vi "Status set defs.vi"(8 "error in (no error)":errorcluster, 11 "MB_TCP in":refnum<class "MB_TCP.lvclass">) -> (0 "error out":errorcluster, 3 "MB_TCP out":refnum<class "MB_TCP.lvclass">)   [LabVIEW 2019, in "MB_TCP.lvclass"]
uses:
  MB_TCP.lvclass
  MB_TCP.lvclass/MB_TCP.ctl
  Eth Status/Eth Status.lvlib
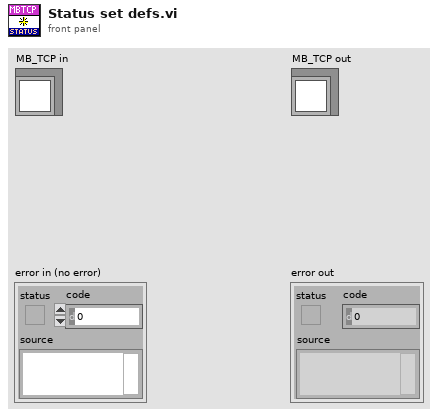
[diagram p1: front panel]
types:
  T1 = typedef "Eth Status.lvlib/ICPCON Status.ctl" = cluster{"Set_state_com":refnum<data-value>, "start":refnum<data-value>, "WrEn":refnum<data-value>, "errors":refnum<data-value>, "connect":refnum<data-value>, "state":refnum<data-value>}
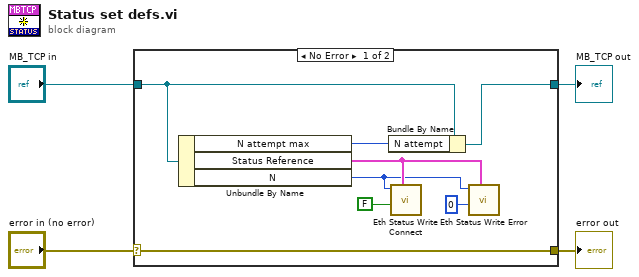
[diagram p0: block diagram]
diagram:
  n1 = case shown="No Error" "error in (no error)" {
    selector: "error in (no error)" -> [w12 w13]
    tunnel: [w12 w13] -> w3
    tunnel: [w5 w14] -> w1
    tunnel: "MB_TCP in" -> [w6 w14]
    frame No Error {
      n2 = Unbundle By Name(w6) -> ("N attempt max"=w11:i32, "Status Reference"=w8:T1, "N"=w7:i32)
      n3 = Bundle By Name(cluster=w6, "N attempt"=w11) -> (w5:refnum<class "MB_TCP.lvclass">)
      n4 = call "Eth Status Write Connect.vi"("Status Reference"=w8, "Connect"=FALSE ("connect"), "N"=w7) -> ()  [unwired: 8 in, 1 out]
      n5 = call "Eth Status Write Error.vi"("Status Reference"=w8, "Errors"=0 ("N attempt max"), "N"=w7) -> ()  [unwired: 8 in, 1 out]
    }
    frame Error {
    }
  }
  "error out" <- w3
  "MB_TCP out" <- w1
